vi "Target_sgl.vi"() -> ()   [LabVIEW 2019]
uses:
  <vilib>/Platform/TimedLoop/XDataNode/timing_clust.ctl
  <vilib>/Platform/TimedLoop/XDataNode/nitl_modes.ctl
  <vilib>/Platform/TimedLoop/XDataNode/wakeup.ctl
  <vilib>/rvi/Emulation/niFpgaSctlEmulationGetInTimedLoop.vi
  <vilib>/rvi/Emulation/niFpgaEmulationReportErrorSimple.vi
  <vilib>/rvi/Emulation/niFpgaGetClockAttributes.vi
  <vilib>/rvi/Emulation/niFpgaCriticalErrorInLSC.vi
  <vilib>/rvi/DataTransferAndStorage/Container/Common/niFpgaContainerExecOnDevCompGetState.vi
  <vilib>/rvi/Emulation/niFpgaEmulationIsFPGAContextNoSignature.vi
  <vilib>/rvi/errors/niFpgaSetErrorForExecOnDevCompSimple.vi
  <vilib>/rvi/eio/common/nirviEmuReportErrorAndStop.vi
  <vilib>/rvi/DataTransferAndStorage/Container/Common/niFpgaContainerGetUniqueNameForEmu.vi
  <vilib>/rvi/FIFO/Fifo_Resource/nirvififoEmulationSetSize.vi
  <vilib>/rvi/FIFO/Fifo_Resource/nirviFifoEmulationQueueMgr.vi
  <instcachedir>/0/nirviFifoEmulationQueueMgr_E5CAEC123FF24DC58D834DCA3CDAA9B5.lvgen/nirviFifoEmulationQueueMgr_E5CAEC123FF24DC58D834DCA3CDAA9B5_005.vi
  <vilib>/rvi/FIFO/Fifo_Resource/nirvififoEmulationDetermineInputValidOut.vi
  <vilib>/rvi/FIFO/Fifo_Resource/nirvififoEmulationCreateLock.vi
  <vilib>/rvi/Emulation/niFpgaProcessEmulError.vi
  <vilib>/rvi/FIFO/Fifo_Resource/nirvififoEmulationObtainLock.vi
  <vilib>/rvi/FIFO/Fifo_Resource/nirvififoEmulationReleaseLock.vi
  <vilib>/rvi/occurrence/nirviWaitOnOccurrenceBase.vi
  <vilib>/rvi/errors/nirviReportUnexpectedCaseInternalError.vi
  <vilib>/rvi/errors/nirviReportUnexpectedCaseInternalError (U32).vi
  <vilib>/Utility/error.llb/Clear Errors.vi
  <vilib>/rvi/interface/RandomDataEmulation/niFpgaRandomDataHandleErrors.vi
  <vilib>/platform/TimedLoop/XDataNode/XDataNode.xnode
  <vilib>/rvi/DataTransferAndStorage/Container/XNode/niFpgaContainer.xnode
  <vilib>/rvi/FIFO/Fifo_Resource/niFpgaFifoEmulationRefIn.vi
  <vilib>/Platform/TimedLoop/XDataNode/XDNodeRunTimeDep.lvlib
panel:
  out "T5":u32 caption="Tick Count(mSec)"
  out "T4":u32 caption="Tick Count(mSec)"
  out "T3":u32 caption="Tick Count(mSec)"
  out "T2":u32 caption="Tick Count(mSec)"
  out "T1":u32 caption="Tick Count(mSec)"
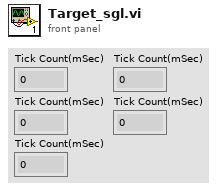
[diagram p1: front panel]
types:
  T1 = typedef "XDNodeRunTimeDep.lvlib/timing_clust.ctl" = cluster{"Expected End [f-1]":u64, "Actual End [f-1]":u64, "Finished Late? [f-1]":bool, "Expected End [i-1]":u64, "Actual End [i-1]":u64, "Finished Late? [i-1]":bool, "Expected Start [i]":u64, "Actual Start [i]":u64, "Expected Start [f]":u64, "Actual Start [f]":u64, "Source Name":string, "Structure Name":string, "Period":i64, "Deadline":i64, "Offset":i64, "Start":i64, "Priority":i32, "Timeout":i32, "Mode":T2, "Wakeup Reason":T3, "Error":errorcluster, "Source Type":string, "Secondary Source Type":string, "Global End Time":u64, "Global Start Time":u64, "Frame Duration":u64, "Iteration Duration":u64, "Assigned CPU":i32, "I/O Scan Engine Mode":u32}
  T2 = typedef "XDNodeRunTimeDep.lvlib/nitl_modes.ctl" = enum32{"No Change", "Process missed periods, maintain original phase", "Discard missed periods, maintain original phase", "Process missed periods, ignore original phase", "Discard missed periods, ignore original phase"}
  T3 = typedef "XDNodeRunTimeDep.lvlib/wakeup.ctl" = enum32{"Normal", "Aborted", "Asynchronous wakeup", "Timing source error", "Timed loop error", "Timeout"}
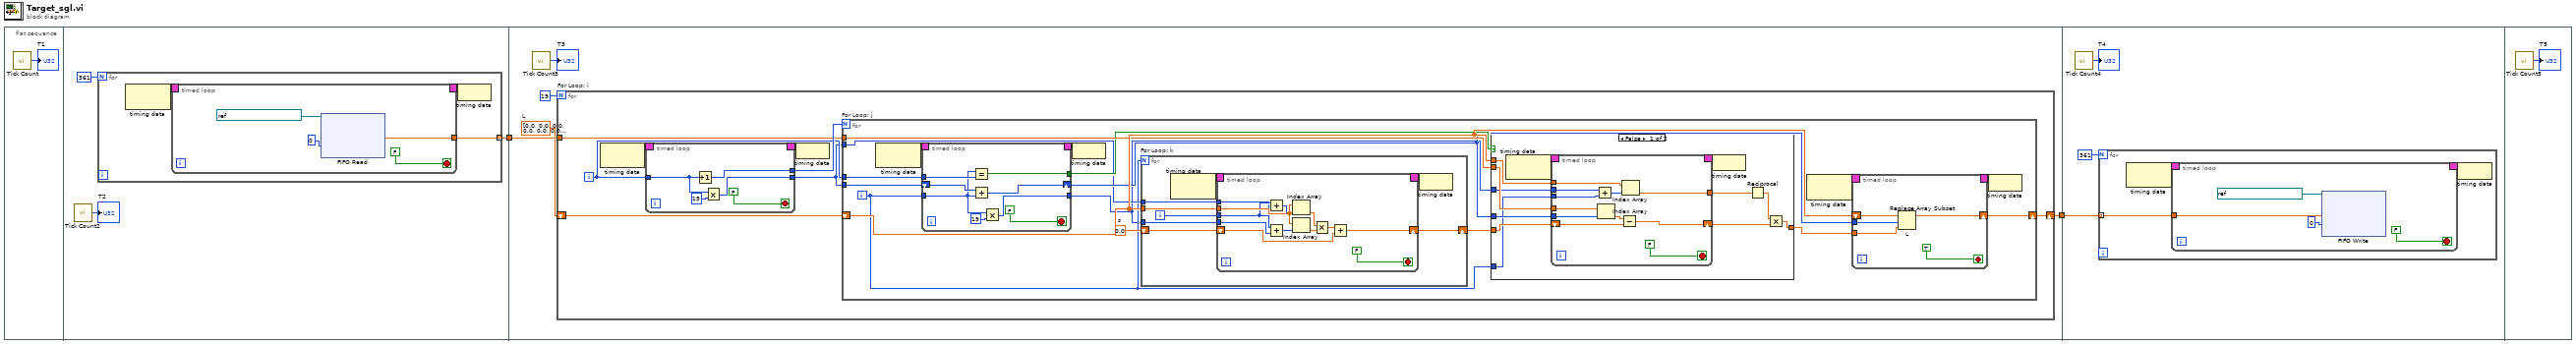
[diagram p0: block diagram]
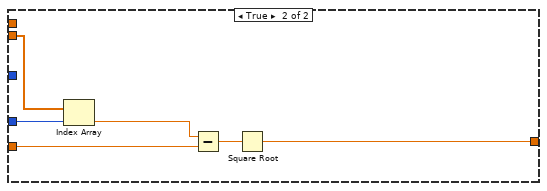
[diagram p2: hidden frame]
diagram:
  n1 = flat-sequence {
    tunnel: [w5] -> w2
    tunnel: w2 -> [w22]
    tunnel: [w21] -> w1
    tunnel: w1 -> [w136]
    frame #0 {
      n2 = call "Tick Count"() -> ("Tick Count(mSec)"=→"T1":u32)
    }
    frame #1 {
      n3 = call "Tick Count2"() -> ("Tick Count(mSec)"=→"T2":u32)
      n4 = for {
        N: 361 -> [_]
        tunnel: [w9] -> w5 mode=indexing
        n5 = node-c288() -> (w8:T1)  [unwired: 1 in]
        n6 = timed-loop {
          timing: w8 -> [_]
          timing-out: [_] -> w7
          tunnel: [w12] -> w9
          stop <- FALSE stop-if-true
          n7 = xnode ("FIFO Read")("Timeout"=0, "FIFO In"=refnum<k21> "FIFO-host-to-Cholesky") -> ("Element"=w12:sgl)  [unwired: 2 out]
        }
        n8 = node-c288(w7) -> ()
      }
    }
    frame #2 {
      w20 = sgl[] [0.0, 0.0, 0.0, 0.0, 0.0, 0.0, 0.0, 0.0, 0.0, 0.0, 0.0, 0.0, 0.0, 0.0, 0.0, 0.0, 0.0, 0.0, 0.0, 0.0, 0.0, 0.0, 0.0, 0.0, 0.0, 0.0, 0.0, 0.0, 0.0, 0.0, 0.0, 0.0, 0.0, 0.0, 0.0, 0.0, 0.0, 0.0, 0.0, 0.0, 0.0, 0.0, 0.0, 0.0, 0.0, 0.0, 0.0, 0.0, 0.0, 0.0, 0.0, 0.0, 0.0, 0.0, 0.0, 0.0, 0.0, 0.0, 0.0, 0.0, 0.0, 0.0, 0.0, 0.0, 0.0, 0.0, 0.0, 0.0, 0.0, 0.0, 0.0, 0.0, 0.0, 0.0, 0.0, 0.0, 0.0, 0.0, 0.0, 0.0, 0.0, 0.0, 0.0, 0.0, 0.0, 0.0, 0.0, 0.0, 0.0, 0.0, 0.0, 0.0, 0.0, 0.0, 0.0, 0.0, 0.0, 0.0, 0.0, 0.0, 0.0, 0.0, 0.0, 0.0, 0.0, 0.0, 0.0, 0.0, 0.0, 0.0, 0.0, 0.0, 0.0, 0.0, 0.0, 0.0, 0.0, 0.0, 0.0, 0.0, 0.0, 0.0, 0.0, 0.0, 0.0, 0.0, 0.0, 0.0, 0.0, 0.0, 0.0, 0.0, 0.0, 0.0, 0.0, 0.0, 0.0, 0.0, 0.0, 0.0, 0.0, 0.0, 0.0, 0.0, 0.0, 0.0, 0.0, 0.0, 0.0, 0.0, 0.0, 0.0, 0.0, 0.0, 0.0, 0.0, 0.0, 0.0, 0.0, 0.0, 0.0, 0.0, 0.0, 0.0, 0.0, 0.0, 0.0, 0.0, 0.0, 0.0, 0.0, 0.0, 0.0, 0.0, 0.0, 0.0, 0.0, 0.0, 0.0, 0.0, 0.0, 0.0, 0.0, 0.0, 0.0, 0.0, 0.0, 0.0, 0.0, 0.0, 0.0, 0.0, 0.0, 0.0, 0.0, 0.0, 0.0, 0.0, 0.0, 0.0, 0.0, 0.0, 0.0, 0.0, 0.0, 0.0, 0.0, 0.0, 0.0, 0.0, 0.0, 0.0, 0.0, 0.0, 0.0, 0.0, 0.0, 0.0, 0.0, 0.0, 0.0, 0.0, 0.0, 0.0, 0.0, 0.0, 0.0, 0.0, 0.0, 0.0, 0.0, 0.0, 0.0, 0.0, 0.0, 0.0, 0.0, 0.0, 0.0, 0.0, 0.0, 0.0, 0.0, 0.0, 0.0, 0.0, 0.0, 0.0, 0.0, 0.0, 0.0, 0.0, 0.0, 0.0, 0.0, 0.0, 0.0, 0.0, 0.0, 0.0, 0.0, 0.0, 0.0, 0.0, 0.0, 0.0, 0.0, 0.0, 0.0, 0.0, 0.0, 0.0, 0.0, 0.0, 0.0, 0.0, 0.0, 0.0, 0.0, 0.0, 0.0, 0.0, 0.0, 0.0, 0.0, 0.0, 0.0, 0.0, 0.0, 0.0, 0.0, 0.0, 0.0, 0.0, 0.0, 0.0, 0.0, 0.0, 0.0, 0.0, 0.0, 0.0, 0.0, 0.0, 0.0, 0.0, 0.0, 0.0, 0.0, 0.0, 0.0, 0.0, 0.0, 0.0, 0.0, 0.0, 0.0, 0.0, 0.0, 0.0, 0.0, 0.0, 0.0, 0.0, 0.0, 0.0, 0.0, 0.0, 0.0, 0.0, 0.0, 0.0, 0.0, 0.0, 0.0, 0.0, 0.0, 0.0, 0.0, 0.0, 0.0, 0.0, 0.0, 0.0, 0.0, 0.0, 0.0, 0.0, 0.0, 0.0, 0.0, 0.0, 0.0, 0.0, 0.0, 0.0, 0.0, 0.0, 0.0, 0.0, 0.0]  # L
      n9 = call "Tick Count3"() -> ("Tick Count(mSec)"=→"T3":u32)
      n10 = for "For Loop: i" {
        N: 19 -> [_]
        shift-right: [w28] -> w21
        shift-left: w20 -> [w30]
        tunnel: w22 -> [w27]
        i -> [w26]
        n11 = node-c288() -> (w24:T1)  [unwired: 1 in]
        n12 = timed-loop {
          timing: w24 -> [_]
          timing-out: [_] -> w23
          tunnel: [w35] -> w29
          tunnel: w26 -> [w33]
          tunnel: [w32] -> w25
          stop <- FALSE stop-if-true
          n13 = Increment(x=w33) -> (x+1=w35:i32)
          n14 = Multiply(x=w33, y=19) -> (x*y=w32:i32)
        }
        n15 = node-c288(w23) -> ()
        n16 = for "For Loop: j" {
          N: w29 -> [_]
          tunnel: w26 -> [w52]
          shift-right: [w54] -> w28
          shift-left: w30 -> [w53]
          tunnel: w27 -> [w51]
          tunnel: w25 -> [w45]
          tunnel: w25 -> [w44]
          i -> [w43]
          w56 = sgl 0.0  # s
          n17 = node-c288() -> (w41:T1)  [unwired: 1 in]
          n18 = timed-loop {
            timing: w41 -> [_]
            timing-out: [_] -> w40
            tunnel: w52 -> [w64]
            tunnel: [w63] -> w50
            tunnel: w43 -> [w59]
            tunnel: [w58] -> w42
            shift-right: [w62] -> w48
            shift-left: w45 -> [w61]
            stop <- FALSE stop-if-true
            n19 = Equal?(x=w59, y=w64) -> (x = y?=w63:bool)
            n20 = Add(x=w61, y=w59) -> (x+y=w62:i32)
            n21 = Multiply(x=w59, y=19) -> (x*y=w58:i32)
          }
          n22 = node-c288(w40) -> ()
          n23 = for "For Loop: k" {
            N: w43 -> [_]
            tunnel: w53 -> [w118]
            shift-right: [w116] -> w55
            shift-left: w56 -> [w117]
            tunnel: w44 -> [w114]
            tunnel: w42 -> [w113]
            i -> [w115]
            n24 = node-c288() -> (w112:T1)  [unwired: 1 in]
            n25 = timed-loop {
              timing: w112 -> [_]
              timing-out: [_] -> w111
              tunnel: w118 -> [w129]
              tunnel: w115 -> [w122]
              tunnel: w114 -> [w121]
              tunnel: w113 -> [w120]
              shift-right: [w125] -> w116
              shift-left: w117 -> [w126]
              stop <- FALSE stop-if-true
              n26 = Add(x=w122, y=w121) -> (x+y=w124:i32)
              n27 = Add(x=w122, y=w120) -> (x+y=w123:i32)
              n28 = Index Array(array=w129, index=w124) -> (element=w130:sgl)
              n29 = Index Array(array=w129, index=w123) -> (element=w128:sgl)
              n30 = Multiply(x=w130, y=w128) -> (x*y=w127:sgl)
              n31 = Add(x=w127, y=w126) -> (x+y=w125:sgl)
            }
            n32 = node-c288(w111) -> ()
          }
          n33 = case shown="False" w50 {
            tunnel: w55 -> [w87 w110]
            tunnel: [w86 w108] -> w49
            tunnel: w53 -> [w89 _]
            tunnel: w51 -> [w83 w107]
            tunnel: w48 -> [w82 w106]
            tunnel: w43 -> [w81 _]
            tunnel: w42 -> [w80 _]
            frame False {
              n34 = node-c288() -> (w79:T1)  [unwired: 1 in]
              n35 = timed-loop {
                timing: w79 -> [_]
                timing-out: [_] -> w78
                tunnel: w89 -> [w100]
                tunnel: [w99] -> w88
                tunnel: w83 -> [w96]
                tunnel: w82 -> [w95]
                tunnel: w81 -> [w93]
                tunnel: w80 -> [w91]
                shift-right: [w97] -> w84
                shift-left: w87 -> [w98]
                stop <- FALSE stop-if-true
                n36 = Add(x=w91, y=w93) -> (x+y=w92:i32)
                n37 = Index Array(array=w96, index=w95) -> (element=w94:sgl)
                n38 = Subtract(x=w94, y=w98) -> (x-y=w97:sgl)
                n39 = Index Array(array=w100, index=w92) -> (element=w99:sgl)
              }
              n40 = node-c288(w78) -> ()
              n41 = Reciprocal(x=w88) -> (1/x=w85:sgl)
              n42 = Multiply(x=w85, y=w84) -> (x*y=w86:sgl)
            }
            frame True {
              n43 = Index Array(array=w107, index=w106) -> (element=w105:sgl)
              n44 = Subtract(x=w105, y=w110) -> (x-y=w109:sgl)
              n45 = Square Root(x=w109) -> (sqrt(x)=w108:sgl)
            }
          }
          n46 = node-c288() -> (w47:T1)  [unwired: 1 in]
          n47 = timed-loop {
            timing: w47 -> [_]
            timing-out: [_] -> w46
            tunnel: w49 -> [w71]
            tunnel: w48 -> [w70]
            shift-right: [w73] -> w54
            shift-left: w53 -> [w72]
            stop <- TRUE stop-if-true
            n48 = Replace Array Subset "L"(array=w72, new element=w71, index=w70) -> (w73:sgl[])
          }
          n49 = node-c288(w46) -> ()
        }
      }
    }
    frame #3 {
      n50 = call "Tick Count4"() -> ("Tick Count(mSec)"=→"T4":u32)
      n51 = for {
        N: 361 -> [_]
        tunnel: w136 -> [w140] mode=indexing
        n52 = node-c288() -> (w139:T1)  [unwired: 1 in]
        n53 = timed-loop {
          tunnel: w140 -> [w143]
          timing: w139 -> [_]
          timing-out: [_] -> w138
          stop <- FALSE stop-if-true
          n54 = xnode ("FIFO Write")("Element"=w143, "Timeout"=0, "FIFO In"=refnum<k21> "FIFO-Cholesky-to-host") -> ()  [unwired: 2 out]
        }
        n55 = node-c288(w138) -> ()
      }
    }
    frame #4 {
      n56 = call "Tick Count5"() -> ("Tick Count(mSec)"=→"T5":u32)
    }
  }
